vi "Generate.vi"(8 "error in (no error)":errorcluster, 9 "Message Queue":refnum<queue>, 10 "Advanced Waveform.lvclass In":refnum<class "Advanced Waveform.lvclass">, 11 "Gen Sine in":refnum<class "Gen Sine.lvclass">) -> (0 "error out":errorcluster, 1 "Message Queue Out":refnum<queue>, 2 "Advanced Waveform.lvclass Out":refnum<class "Advanced Waveform.lvclass">, 3 "Gen Sine out":refnum<class "Gen Sine.lvclass">)   [LabVIEW 2011, in "Gen Sine.lvclass"]
uses:
  Gen Sine.lvclass
  Advanced Waveform Class/Advanced Waveform.lvclass
  Message.lvclass
  Display Message/Display Message.lvclass
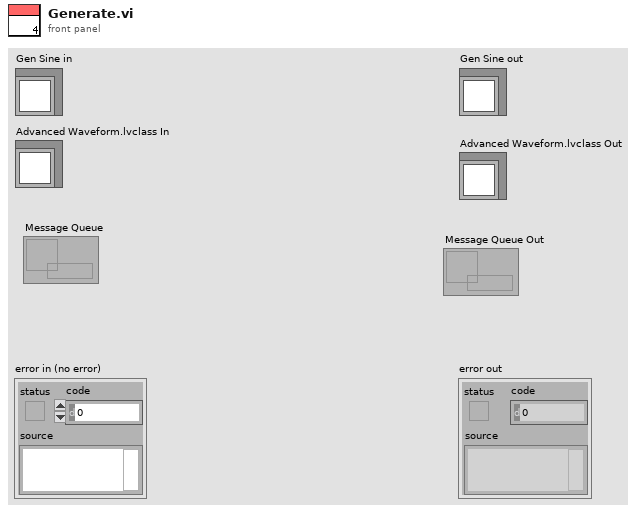
[diagram p1: front panel]
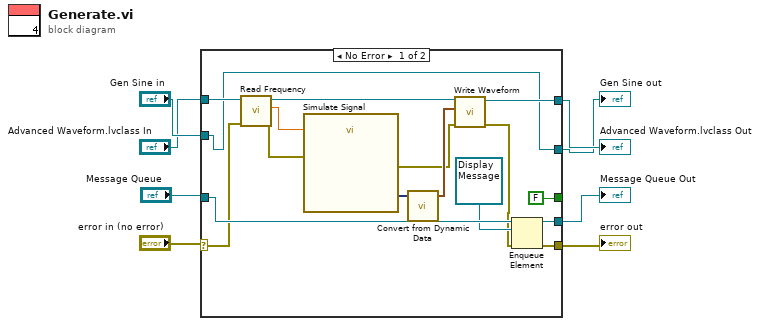
[diagram p0: block diagram]
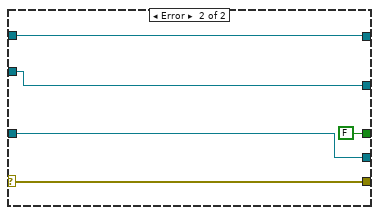
[diagram p2: hidden frame]
diagram:
  n1 = case shown="No Error" "error in (no error)" {
    selector: "error in (no error)" -> [w14 w28]
    tunnel: "Advanced Waveform.lvclass In" -> [w24 w29]
    tunnel: [w21 w29] -> w4
    tunnel: [w10 w25] -> w3
    tunnel: "Message Queue" -> [w18 w26]
    tunnel: [w12 w28] -> w1
    tunnel: [FALSE FALSE] -> _
    tunnel: "Gen Sine in" -> [w10 w25]
    tunnel: [w9 w26] -> w2
    frame No Error {
      n2 = call-dynamic "Read Frequency.vi"("error in (no error)"=w14, "Waveform in"=w24) -> ("error out"=w15:errorcluster, "Frequency"=w23:dbl, "Waveform out"=w22:refnum<class "Advanced Waveform.lvclass">)  [unwired: 7 in]
      n3 = call "Simulate Signal"("Frequency"=w23, "error in (no error)"=w15) -> ("Sine"=w20:dynamicdata, "error out"=w16:errorcluster)  [unwired: 12 in]
      n4 = call "Convert from Dynamic Data"("Dynamic Data Type"=w20) -> ("Waveform"=w19:waveform(dbl))  [unwired: 3 in]
      n5 = call-dynamic "Write Waveform.vi"("error in (no error)"=w16, "Waveform"=w19, "Waveform in"=w22) -> ("error out"=w13:errorcluster, "Waveform out"=w21:refnum<class "Advanced Waveform.lvclass">)  [unwired: 7 in]
      n6 = Enqueue Element(queue=w18, element=refnum<class "Display Message.lvclass"> refnum ("Display Message.lvclass"), error in (no error)=w13) -> (queue out=w9:refnum<queue>, error out=w12:errorcluster)  [unwired: 1 in, 1 out]
    }
    frame Error {
    }
  }
  "error out" <- w1
  "Gen Sine out" <- w3
  "Advanced Waveform.lvclass Out" <- w4
  "Message Queue Out" <- w2
